vi "FilePathInit.vi"(3 "Container State":T3, 4 "Previous State":variant, 5 "Previous Version":T2) -> (2 "Current State":T1)   [LabVIEW 2014, in "FilePathControl.xctl"]
uses:
  <userlib>/CurtinCode/Filexctrl/FilePathControl.xctl
  <userlib>/CurtinCode/Filexctrl/FilePathState.ctl
  <vilib>/_xctls/Container State.ctl
  <vilib>/_xctls/Version.ctl
  <vilib>/_xctls/XControlSupport.lvlib
panel:
  in  "Default Indicator State":T1
  in  "Default Control State":T1
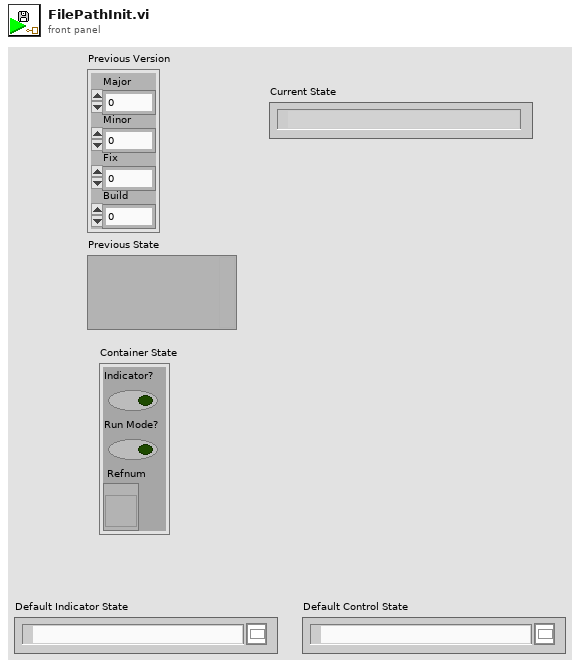
[diagram p1: front panel]
types:
  T1 = typedef "FilePathControl.xctl/FilePathState.ctl" = path
  T2 = typedef "XControlSupport.lvlib/Version.ctl" = cluster{"Major":u16, "Minor":u16, "Fix":u16, "Build":u16}
  T3 = typedef "XControlSupport.lvlib/Container State.ctl" = cluster{"Indicator?":bool, "Run Mode?":bool, " Refnum":refnum<vi>}
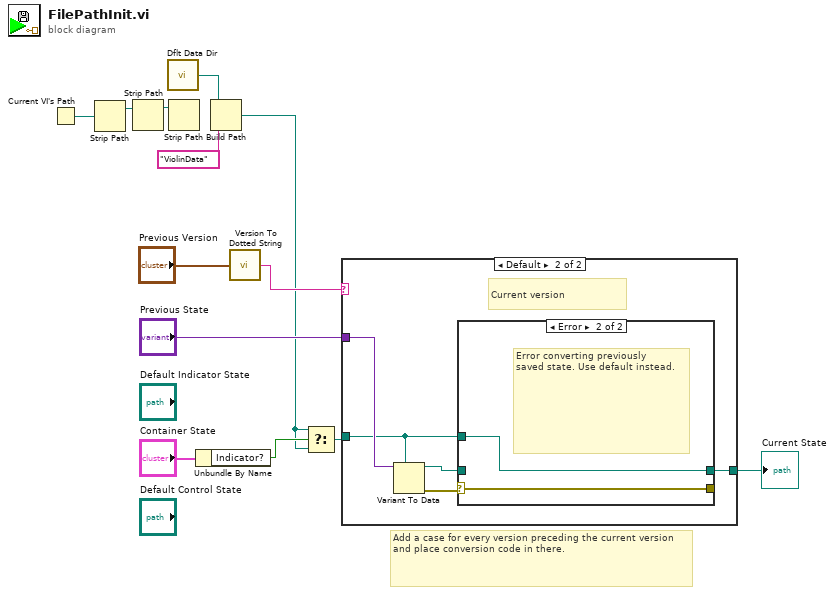
[diagram p0: block diagram]
diagram:
  # "Add a case for every version preceding the current version and place conversion code in there."
  n1 = Current VI's Path() -> (path=w6:path)
  n2 = Strip Path(path=w6) -> (stripped path=w5:path)  [unwired: 1 out]
  n3 = Strip Path(path=w5) -> (stripped path=w4:path)  [unwired: 1 out]
  n4 = call <vilib>:"Dflt Data Dir.vi"() -> ("App:Default Data Directory"=w1:path)
  n5 = Strip Path(path=w4) -> ()  [unwired: 2 out]
  n6 = Unbundle By Name("Container State") -> ("Indicator?"=w10:bool)
  n7 = Build Path(base path=w1, name or relative path="ViolinData") -> (appended path=w2:path)
  n8 = call <vilib>:"Version To Dotted String.vi"("Version"="Previous Version") -> ("String Version"=w7:string)
  n9 = Select(t=w2, s=w10, f=w2) -> (s? t:f=w9:path)
  n10 = case shown="Default" w7 {
    tunnel: "Previous State" -> [_ w19]
    tunnel: [w14 w15] -> w12
    tunnel: w9 -> [w14 w16]
    frame "0.0.0.0" {
      # "Just created, use default state"
    }
    frame Default {
      # "Current version"
      n11 = Variant To Data(type=w16, Variant=w19) -> (data=w17:path, error out=w18:errorcluster)  [unwired: 1 in]
      n12 = case shown="Error" w18 {
        selector: w18 -> [w21 w22]
        tunnel: w17 -> [w20 _]
        tunnel: [w20 w23] -> w15
        tunnel: w16 -> [_ w23]
        tunnel: [w21 w22] -> _
        frame No Error {
        }
        frame Error {
          # "Error converting previously \nsaved state. Use default instead."
        }
      }
    }
  }
  "Current State" <- w12
